vi "LN_SetNextNodeRef.vi"(2 "InputNextNodeRef":refnum<data-value>, 3 "InputListNode":refnum<class "ListNode.lvclass">) -> (1 "OutputListNode":refnum<class "ListNode.lvclass">)   [LabVIEW 2014, in "ListNode.lvclass"]
uses:
  ListNode.lvclass
  ListNodeVirtual.lvclass
  ListNode.lvclass/ListNode.ctl
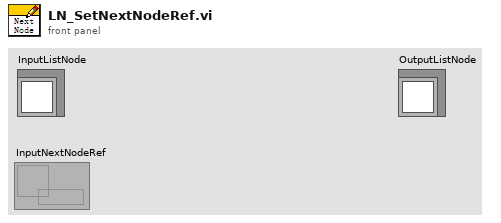
[diagram p1: front panel]
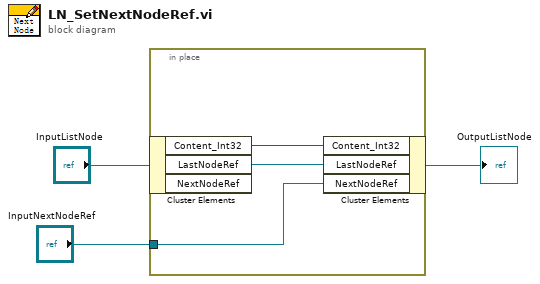
[diagram p0: block diagram]
diagram:
  n1 = in-place {
    in-place-border: "InputNextNodeRef" -> [w4]
    n2 = in-place-cluster #1("InputListNode") -> ("Content_Int32"=w6:i32, "LastNodeRef"=w5:refnum<data-value>)  [unwired: 1 out]
    n3 = in-place-cluster #1("Content_Int32"=w6, "LastNodeRef"=w5, "NextNodeRef"=w4) -> (→"OutputListNode":refnum<class "ListNode.lvclass">)
  }
